vi "AbortGeneration.vi"(8 "error in (no error)":errorcluster, 11 "ClassIn":refnum<class "NiPxi6733.lvclass">) -> (0 "error out":errorcluster, 3 "ClassOut":refnum<class "NiPxi6733.lvclass">)   [LabVIEW 2014, in "FGenPlugins.lvlib" / "NiPxi6733.lvclass"]
uses:
  NiPxi6733.lvclass
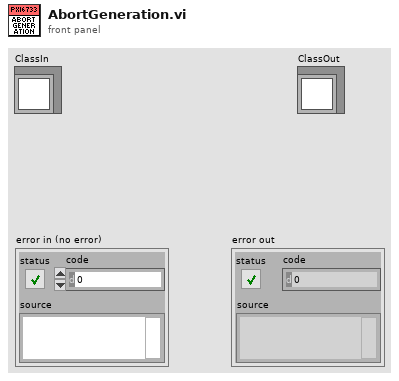
[diagram p1: front panel]
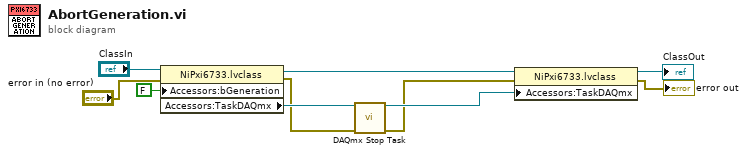
[diagram p0: block diagram]
diagram:
  n1 = property class="NiPxi6733.lvclass"(reference="ClassIn", error in="error in (no error)", "Accessors:bGeneration"=FALSE ("bGeneration")) -> (reference out=w7:refnum<class "NiPxi6733.lvclass">, error out=w2:errorcluster, "Accessors:TaskDAQmx"=w8:refnum<k21>)
  n2 = call <vilib>:"DAQmx Stop Task.vi"("task/channels in"=w8, "error in"=w2) -> ("task out"=w6:refnum<k21>, "error out"=w1:errorcluster)  [unwired: 12 in]
  n3 = property class="NiPxi6733.lvclass"(reference=w7, error in=w1, "Accessors:TaskDAQmx"=w6) -> (reference out=→"ClassOut":refnum<class "NiPxi6733.lvclass">, error out=→"error out":errorcluster)
